vi "Configuration UI.vi"(0 "Engine":refnum<k7>, 5 "Data In":T1, 7 "Sequence Context In":refnum<k7>, 11 "error in (no error)":errorcluster) -> (4 "Engine out":refnum<k7>, 6 "Data Out":T1, 8 "Changed":bool, 15 "error out":errorcluster)   [LabVIEW 2019, in "STS_LTRV.lvlib"]
uses:
  STS_LTRV.lvlib
  TypeDefs/Config UI Data Type.ctl
  SimpleTextPlugin.llb/SimpleTextRpt - TestStand - Start Modal Dialog (Engine).vi
  SimpleTextPlugin.llb/SimpleTextRpt - TestStand - End Modal Dialog (Engine).vi
  SimpleTextPlugin.llb/SimpleTextRpt - Set Cursor (Icon Pict).vi
panel:
  in  "Max UUT Records to Store":u32=4 min=4
  in  "TS_HELP":bool
  in  "TS_CANCEL":bool
  in  "TS_OK":bool
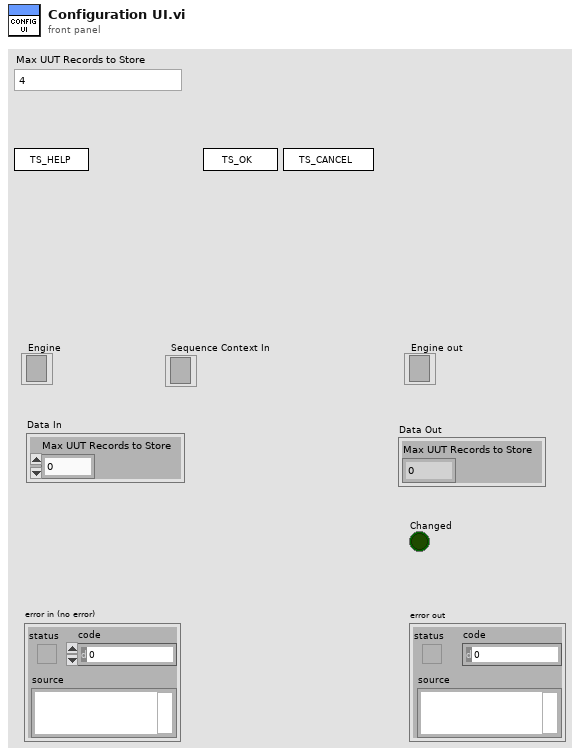
[diagram p1: front panel]
types:
  T1 = typedef "STS_LTRV.lvlib/Config UI Data Type.ctl" = cluster{"Max UUT Records to Store":u32}
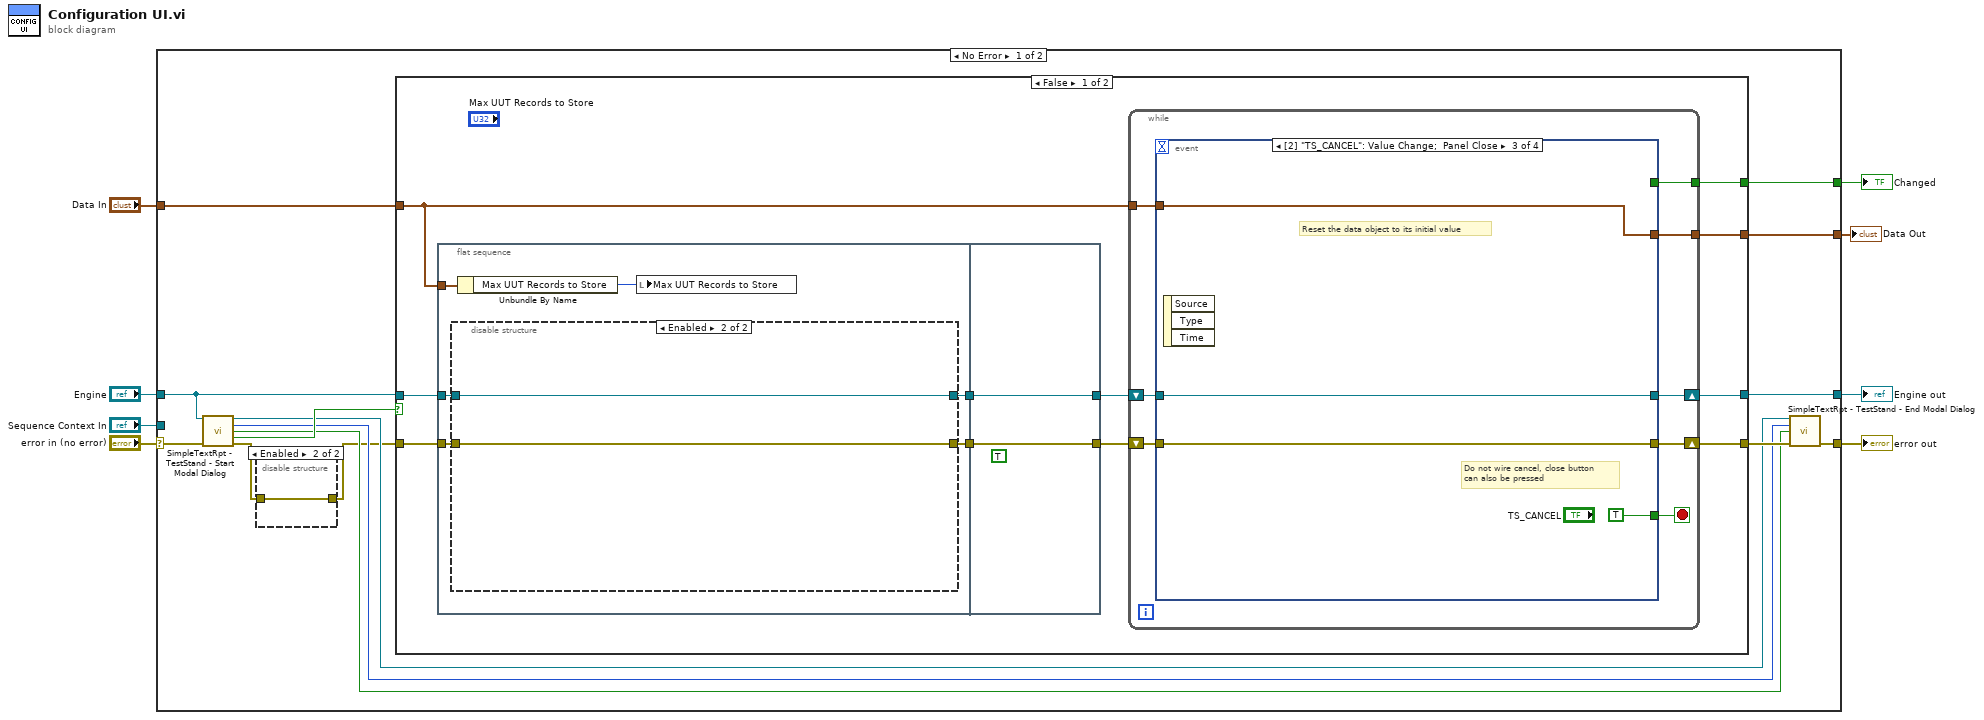
[diagram p0: block diagram]
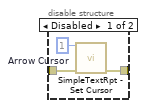
[diagram p2: hidden frame]
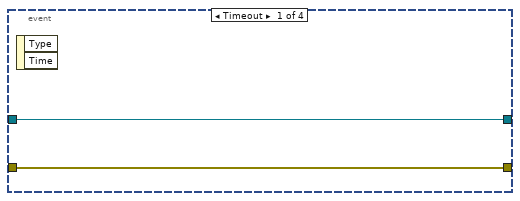
[diagram p3: hidden frame]
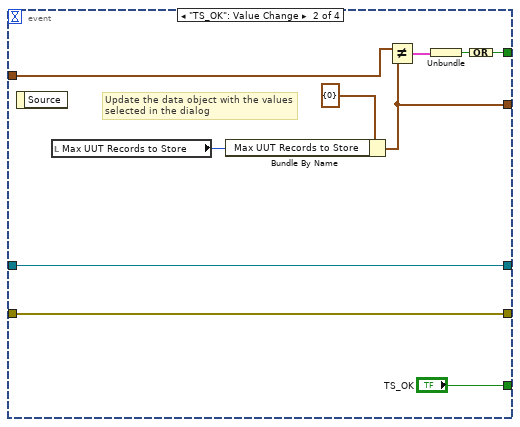
[diagram p4: hidden frame]
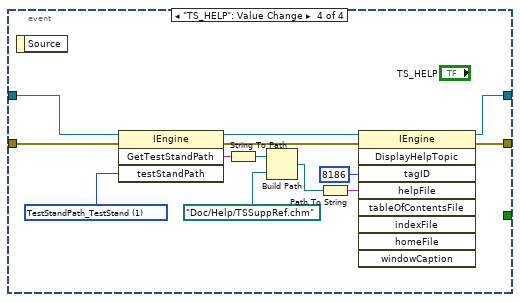
[diagram p5: hidden frame]
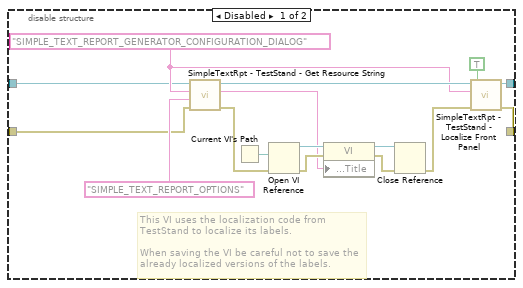
[diagram p6: hidden frame]
diagram:
  n1 = case shown="No Error" "error in (no error)" {
    selector: "error in (no error)" -> [w14 w106]
    tunnel: "Data In" -> [w22 w104]
    tunnel: [w19 w106] -> w7
    tunnel: [w15 w105] -> w3
    tunnel: [w16 _] -> w5
    tunnel: "Engine" -> [w12 w105]
    tunnel: "Sequence Context In" -> [_ _]
    tunnel: [w9 w104] -> w1
    frame No Error {
      n2 = call-poly "SimpleTextRpt - TestStand - Start Modal Dialog.vi"("Engine in"=w12, "error in (no error)"=w14) -> ("Engine out"=w13:refnum<k7>, "Modal ID"=w18:i32, "VI Originally Open"=w17:bool, "Should Abort"=w21:bool, "error out"=w11:errorcluster)  [unwired: 2 in, 7 out]
      n3 = disable-structure shown="Enabled" {
        disable-tunnel: w11 -> [w25 w26]
        disable-tunnel: [w24 w26] -> w10
        frame Disabled {
          w23 = u16 1  # Arrow Cursor
          n4 = call-poly "SimpleTextRpt - Set Cursor.vi"("error in (no error)"=w25, "icon"=w23) -> ("error out"=w24:errorcluster)  [unwired: 8 in, 1 out]
        }
        frame Enabled {
        }
      }
      n5 = case shown="False" w21 {
        tunnel: [w37 w103] -> w20
        tunnel: w22 -> [w35 w101]
        tunnel: w12 -> [w31 w102]
        tunnel: w10 -> [w29 w103]
        tunnel: [w34 _] -> w16
        tunnel: [w30 w102] -> w15
        tunnel: [w27 w101] -> w9
        frame False {
          n6 = flat-sequence {
            tunnel: w35 -> [w79]
            tunnel: w31 -> [w77]
            tunnel: [w80] -> w33
            tunnel: [w78] -> w32
            tunnel: w29 -> [w76]
            tunnel: [w100] -> w36
            tunnel: w33 -> [w100]
            tunnel: w32 -> [w99]
            tunnel: [w99] -> w28
            frame #0 {
              n7 = disable-structure shown="Enabled" {
                disable-tunnel: [w95 w97] -> w80
                disable-tunnel: [w94 w98] -> w78
                disable-tunnel: w77 -> [w82 w97]
                disable-tunnel: w76 -> [w81 w98]
                frame Disabled {
                  w88 = "SIMPLE_TEXT_REPORT_GENERATOR_CONFIGURATION_DIALOG" ("Category")
                  # "This VI uses the localization code from \nTestStand to localize its labels.\n\nWhen saving the VI be careful not to save the \nalready localized versions of the labels."
                  n8 = call "SimpleTextRpt - TestStand - Get Resource String.vi"("error in (no error)"=w81, "Symbol"="SIMPLE_TEXT_REPORT_OPTIONS", "Category"=w88, "Engine Reference In"=w82) -> ("error out"=w86:errorcluster, "Resource String"=w87:string, "Engine Reference Out"=w89:refnum<k7>)  [unwired: 4 in, 1 out]
                  n9 = Current VI's Path() -> (path=w93:path)
                  n10 = Open VI Reference(vi path=w93, error in (no error)=w86) -> (vi reference=w91:refnum<vi>, error out=w92:errorcluster)  [unwired: 4 in]
                  n11 = property class="VI"(reference=w91, error in=w92, "Front Panel.Title"=w87) -> (reference out=w83:refnum<vi>, error out=w90:errorcluster)
                  n12 = Close Reference(reference=w83, error in (no error)=w90) -> (error out=w84:errorcluster)
                  n13 = call "SimpleTextRpt - TestStand - Localize Front Panel.vi"("Engine Reference In"=w89, "Category"=w88, "error in (no error)"=w84, "Localize Free Labels (False)"=TRUE) -> ("Engine Reference Out"=w95:refnum<k7>, "error out"=w94:errorcluster)  [unwired: 1 in, 4 out]
                }
                frame Enabled {
                }
              }
              n14 = Unbundle By Name(w79) -> ("Max UUT Records to Store"=w75:u32)
              n15 = local write "Max UUT Records to Store"(w75) -> ()
            }
            frame #1 {
              (unwired) TRUE ("Selected")
            }
          }
          n16 = while {
            tunnel: w35 -> [w42]
            shift-right: [w44] -> w37
            shift-left: w28 -> [w43]
            shift-right: [w40] -> w30
            shift-left: w36 -> [w41]
            tunnel: [w39] -> w34
            tunnel: [w38] -> w27
            stop <- w45 stop-if-true
            n17 = event shown="[2] \"TS_CANCEL\": Value Change;  Panel Close" {
              selector: _ -> [_ _ _ _]
              dyn-events: _ -> [_ _ _ _]
              timeout: _ -> [_ _ _ _]
              tunnel: [_ "TS_OK" TRUE ("TS_OK") _] -> w45
              tunnel: [w47 w56 w61 w73] -> w44
              tunnel: w43 -> [w47 w56 w61 w69]
              tunnel: w42 -> [_ w54 w58 _]
              tunnel: w41 -> [w46 w55 w60 w71]
              tunnel: [w46 w55 w60 w72] -> w40
              tunnel: [_ w51 _ _] -> w39
              tunnel: [_ w48 w58 _] -> w38
              event Timeout {
                n18 = event-data() -> ()  [unwired: 3 out]
              }
              event "TS_OK": Value Change {
                # "Update the data object with the values \nselected in the dialog"
                n19 = event-data() -> ()  [unwired: 2 out]
                n20 = local read "Max UUT Records to Store"() -> (w49:u32)
                n21 = Bundle By Name(cluster=T1 {"Max UUT Records to Store"=0} ("Data In"), "Max UUT Records to Store"=w49) -> (w48:T1)
                n22 = Not Equal?(x=w54, y=w48) -> (x != y?=w53:cluster{"Max UUT Records to Store":bool})
                n23 = Unbundle(w53) -> ("Max UUT Records to Store"=w52:bool)
                n24 = Compound Arithmetic op=OR(w52) -> (w51:bool)
              }
              event "TS_CANCEL": Value Change; Panel Close {
                # "Do not wire cancel, close button\ncan also be pressed"
                # "Reset the data object to its initial value"
                n25 = event-data() -> ()  [unwired: 4 out]
              }
              event "TS_HELP": Value Change {
                w67 = 1 items=["TestStandPath_TestStand"=1, "TestStandPath_Bin"=2, "TestStandPath_Config"=3, "TestStandPath_Public"=4, "TestStandPath_CommonAppData"=5, "TestStandPath_LocalAppData"=6, "TestStandPath_PublicComponents"=7, "TestStandPath_NIComponents"=8, "TestStandPath_Temp"=9] ("testStandPath")
                n26 = event-data() -> ()  [unwired: 2 out]
                n27 = invoke class="IEngine" method="GetTestStandPath"(reference=w71, error in=w69, "testStandPath"=w67) -> (reference out=w70:refnum<k7>, error out=w68:errorcluster, "GetTestStandPath"=w65:string)  [unwired: 1 in, 1 out]
                n28 = String To Path(string=w65) -> (path=w66:path)
                n29 = Build Path(base path=w66, name or relative path=path "Doc/Help/TSSuppRef.chm") -> (appended path=w64:path)
                n30 = Path To String(path=w64) -> (string=w62:string)
                n31 = invoke class="IEngine" method="DisplayHelpTopic"(reference=w70, error in=w68, "tagID"=8186, "helpFile"=w62) -> (reference out=w72:refnum<k7>, error out=w73:errorcluster)  [unwired: 5 in, 7 out]
              }
            }
          }
        }
        frame True {
        }
      }
      n32 = call-poly "SimpleTextRpt - TestStand - End Modal Dialog.vi"("Engine"=w13, "Modal ID"=w18, "VI Originally Open"=w17, "error in (no error)"=w20) -> ("error out"=w19:errorcluster)  [unwired: 1 in, 10 out]
    }
    frame Error {
    }
  }
  "error out" <- w7
  "Changed" <- w5
  "Engine out" <- w3
  "Data Out" <- w1
